vi "New Experiment.vi"(8 "error in (no error)":errorcluster, 9 "Experiment File Extension":string, 10 "Experiment Name in":string, 11 "Experiment Location in":path) -> (0 "error out":errorcluster, 1 "Experiment File Cluster":T1, 2 "Experiment Name out":string, 3 "Experiment Location out":path, 4 "cancelled":bool, 5 "Experiment filename out":string)   [LabVIEW 2020, in "Experiment Manager.lvlib"]
uses:
  Experiment Manager.lvlib
  Experiment File/Experiment File Cluster.ctl
  Plugin Servers/Controller/Minimal Controller Cluster.ctl
  Plugin Servers/Parameter to Hardware Map/Minimal Map.ctl
  Plugin Servers/Parameter to Hardware Map/Minimal Pair Cluster.ctl
  Experiment File/Experiment File.lvlib
  Plugin Servers/Controller/Generic Plugin.lvclass
  Plugin Servers/Parameter to Hardware Map/Parameter to Hardware Map.lvclass
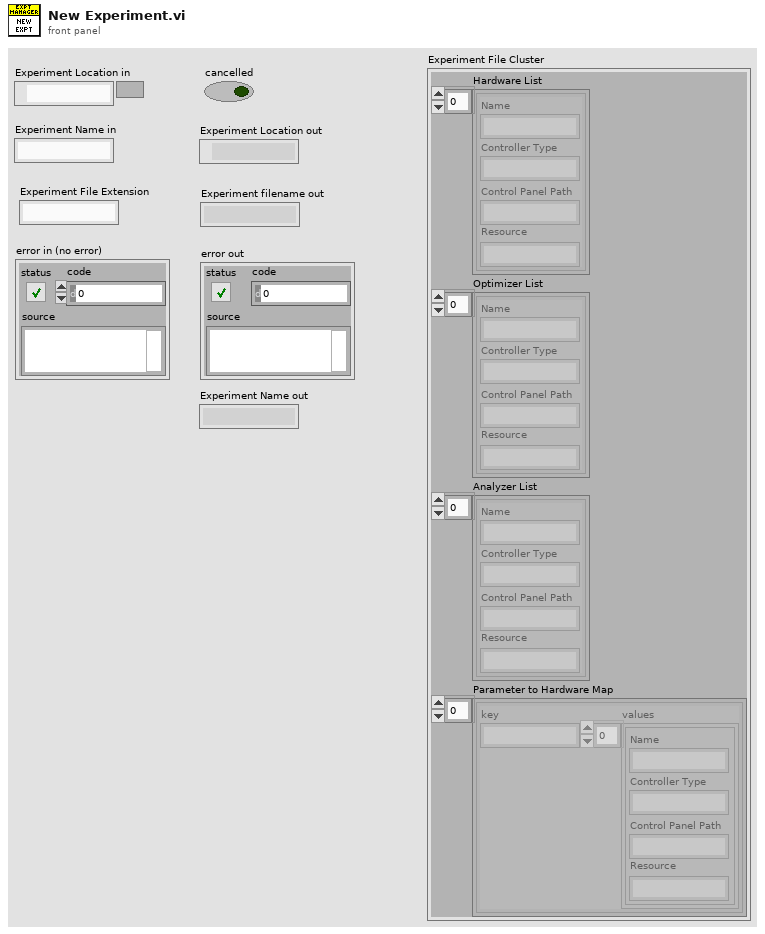
[diagram p1: front panel]
types:
  T1 = typedef "Experiment File.lvlib/Experiment File Cluster.ctl" = cluster{"Hardware List":T2[], "Optimizer List":T2[], "Analyzer List":T2[], "Parameter to Hardware Map":T3}
  T2 = typedef "Generic Plugin.lvclass/Minimal Controller Cluster.ctl" = cluster{"Name":string, "Controller Type":string, "Control Panel Path":string, "Resource":string}
  T3 = typedef "Parameter to Hardware Map.lvclass/Minimal Map.ctl" = T4[]
  T4 = typedef "Parameter to Hardware Map.lvclass/Minimal Pair Cluster.ctl" = cluster{"key":string, "values":T2[]}
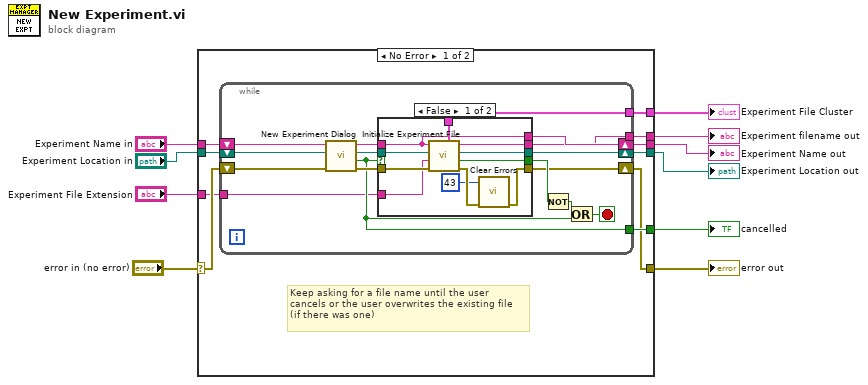
[diagram p0: block diagram]
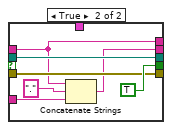
[diagram p2: hidden frame]
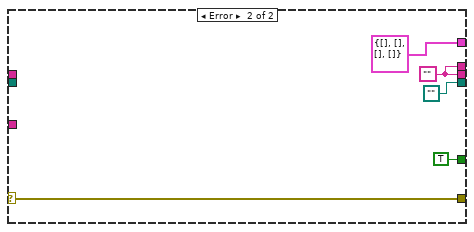
[diagram p3: hidden frame]
diagram:
  n1 = case shown="No Error" "error in (no error)" {
    selector: "error in (no error)" -> [w13 w59]
    tunnel: "Experiment Location in" -> [w20 _]
    tunnel: [w19 path ""] -> w9
    tunnel: [w18 w55] -> w2
    tunnel: [w17 TRUE ("cancelled")] -> w8
    tunnel: [w16 w59] -> w7
    tunnel: [w15 T1 {"Hardware List"=[], "Optimizer List"=[], "Analyzer List"=[], "Parameter to Hardware Map"=[]} ("Experiment File Cluster")] -> w6
    tunnel: "Experiment Name in" -> [w14 _]
    tunnel: [w12 w55] -> w3
    tunnel: "Experiment File Extension" -> [w11 _]
    frame No Error {
      # "Keep asking for a file name until the user\ncancels or the user overwrites the existing file\n(if there was one)"
      n2 = while {
        shift-right: [w33] -> w19
        shift-left: w20 -> [w32]
        shift-right: [w23] -> w18
        shift-left: w14 -> [w24]
        shift-right: [w29] -> w16
        shift-left: w13 -> [w31]
        tunnel: [w28] -> w15
        tunnel: [w25] -> w17
        tunnel: [w22] -> w12
        tunnel: w11 -> [w21]
        stop <- w27 stop-if-true
        n3 = call "New Experiment Dialog.vi"("error in (no error)"=w31, "Experiment Location"=w32, "Experiment Name"=w24) -> ("error out"=w30:errorcluster, "cancelled"=w25:bool, "Project Directory out"=w36:path, "Project Name out"=w35:string)  [unwired: 5 in]
        n4 = case shown="False" w25 {
          tunnel: w36 -> [w47 w53]
          tunnel: w35 -> [w38 w50]
          tunnel: [w46 TRUE ("cancelled")] -> w34
          tunnel: [w45 w51] -> w22
          tunnel: [w44 w53] -> w33
          tunnel: w30 -> [w43 w52]
          tunnel: [w40 w52] -> w29
          tunnel: [w42 _] -> w28
          tunnel: [w38 w50] -> w23
          tunnel: w21 -> [w37 w49]
          frame False {
            n5 = call "Initialize Experiment File.vi"("error in (no error)"=w43, "Experiment File Extension"=w37, "Experiment Directory"=w47, "Experiment Name"=w38) -> ("error out"=w41:errorcluster, "cancelled"=w46:bool, "Experiment Location out"=w44:path, "Experiment File Name out"=w45:string, "Experiment File Cluster"=w42:T1)  [unwired: 3 in]
            n6 = call <vilib>:"Clear Errors.vi"("error in (no error)"=w41, "specific error code to clear (0: all)"=43) -> ("error out"=w40:errorcluster)  [unwired: 4 in, 1 out]
          }
          frame True {
            n7 = Concatenate Strings(w50, "." ("string"), w49) -> (w51:string)
          }
        }
        n8 = Not(x=w34) -> (.not. x?=w26:bool)
        n9 = Or(x=w26, y=w25) -> (x .or. y?=w27:bool)
      }
    }
    frame Error {
      w55 = ""
    }
  }
  "Experiment Location out" <- w9
  "Experiment filename out" <- w3
  "cancelled" <- w8
  "error out" <- w7
  "Experiment File Cluster" <- w6
  "Experiment Name out" <- w2
